vi "GenAppMainResize.vi"() -> ()   [LabVIEW 2018]
doc: "DESCRIPTION\nGeneral Application \n\nVERSION\nD1:00\nFirst Release To customer\nDD/MM/YYYY\n\nTemplate D2:01\nMade lighter and simpler\n14-04-2020"
uses:
  SubVIs/Controls/SetupModeState.ctl
  <vilib>/event_ctls.llb/eventsource.ctl
  SubVIs/Controls/DisplayQCommand.ctl
  SubVIs/Controls/QueueCommand.ctl
  SubVIs/Controls/DisplayMessage.ctl
  SubVIs/Controls/Transition.ctl
  SubVIs/utilities/Error/ErrorCommand.ctl
  SubVIs/Controls/Tab.ctl
  SubVIs/Controls/StateMessage.ctl
  SubVIs/Error/ErrorMessage.ctl
  SubVIs/utilities/Config/System Config Data Manager Parameter.ctl
  SubVIs/utilities/Config/ConfigCommand.ctl
panel:
  out "Time":string
  out "Version":string
  out "State":T1=enum."Initialising"
  out "Error":string
  out "ErrorIndicator":bool
  in  "ViewError":bool
  in  "Main Screen Tabs":enum32{"Main Screen"}(tab)
  out "Tab Control":T2(tab)
  out "ConfigdB path":path
  in  "ErrorLog":i32(listbox)
  in  "ButtonTabs":enum32{"Normal", "Error"}(tab)
  in  "Clear Alarm":bool
  in  "ErrorLog 2":bool
  in  "Home Button":bool
  in  "Error Loop":enum16{"Event Loop", "UI Q Loop", "State Loop"}(ring)
  in  "Generate Error":bool
  out "ErrorHandlingLoop":i32
  out "StateMachineLoop":i32
  out "UILoop":i32
  out "EventLoop":i32
  in  "Enter Password":string
  out "EngMode?":bool
  out "Status":string
  in  "Source":T3 items=["LabVIEW UI"=0, "ActiveX"=1, "User Event"=25]
  in  "exit":bool
  in  "Stop":bool
  in  "Start":bool
  # "GenAppMainResize"
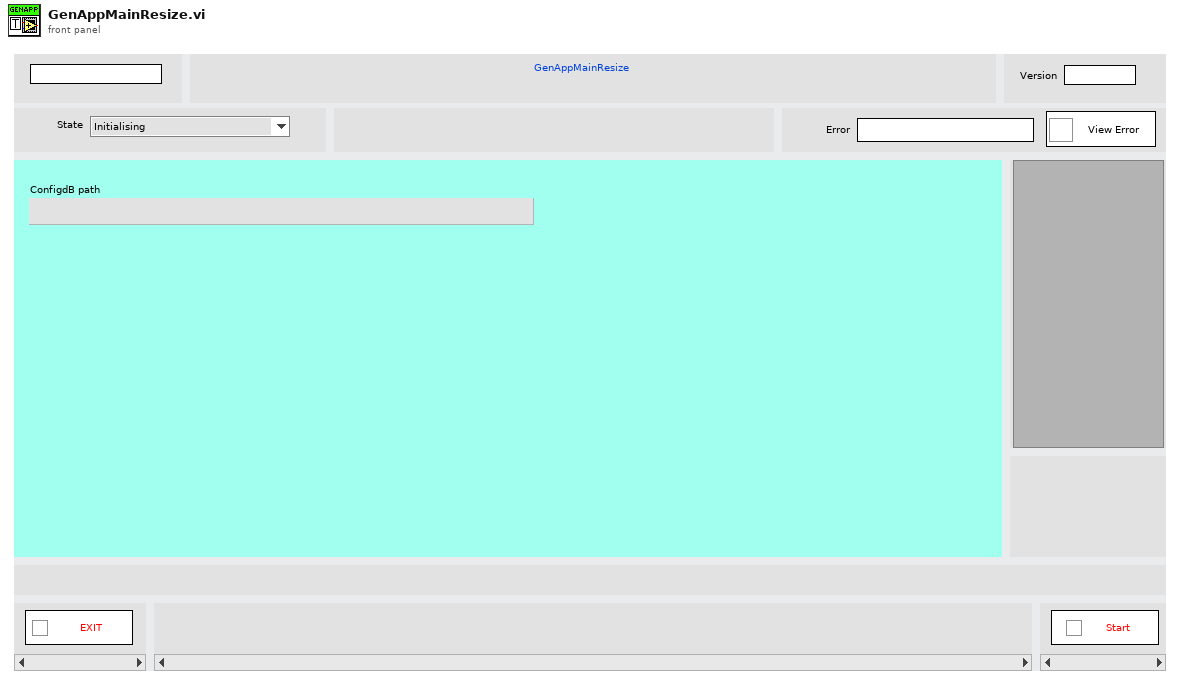
[diagram p1: front panel]
types:
  T1 = typedef "SetupModeState.ctl" = enum16{"No State - Error", "Initialising", "Idling", "Running", "Erroring", "Exiting"}
  T2 = enum32{"Welcome Screen", "Eng Set Up", "Oppo Run Screen", "Eng Run Screen", "Test Report Screen", "Error"}
  T3 = typedef "eventsource.ctl" = u32
  T4 = typedef "DisplayQCommand.ctl" = enum16{"No Command - Error", "Initialise", "Get Q Reference", "Add Item to Bottom", "Add Item to Top", "Flush Q", "Dequeue", "Peek Next Element", "Close"}
  T5 = typedef "QueueCommand.ctl" = enum16{"No Command - Error", "Initialise", "Add to Bottom", "Add To Top", "Get Ref", "Close"}
  T6 = typedef "ErrorCommand.ctl" = enum16{"No Command - Error", "Set to Dev Mode", "Set To Released Mode", "Set Error", "Log Error", "Throw Error", "Log & Throw Error", "Set Error Timed"}
  T7 = enum32{"invalid app kind", "Development System", "Run Time System", "Student Edition", "Embedded LabVIEW", "Evaluation", "Custom"}
  T8 = typedef "DisplayMessage.ctl" = enum16{"No Message - Ignore", "Display Message", "Set Tab", "Set Status", "Add Error Message", "Clear Error History", "Generate Error", "Set Idling Display", "Set Running Display", "Stop"}
  T9 = typedef "ErrorMessage.ctl" = enum16{"No Message - Ignore", "Display Message", "Stop"}
  T10 = typedef "StateMessage.ctl" = cluster{"Transition":T11, "variant":variant}
  T11 = typedef "Transition.ctl" = enum16{"No Transition - Error", "Initialise", "Login", "Authenticate", "Log on Fail", "Login Success", "Logout", "Generate Error", "Start", "Stop", "Exit"}
  T12 = typedef "ConfigCommand.ctl" = enum16{"No Command - Error", "Initialise Config SQLite", "Save Config", "Get Key", "Set Key", "Update Key", "Get Latest Config Data", "Get Config Data for Version", "Get Default Config Data"}
  T13 = typedef "System Config Data Manager Parameter.ctl" = enum16{"Eng Password", "DSN Connection", "User Password", "RunStatus", "InitialDataPath", "helpFilePath", "ErrorFilepath", "DatalogPath", "Hello"}
  T14 = typedef "Tab.ctl" = enum32{"Welcome Screen", "Eng Set Up", "Oppo Run Screen", "Eng Run Screen", "Test Report Screen", "Error"}
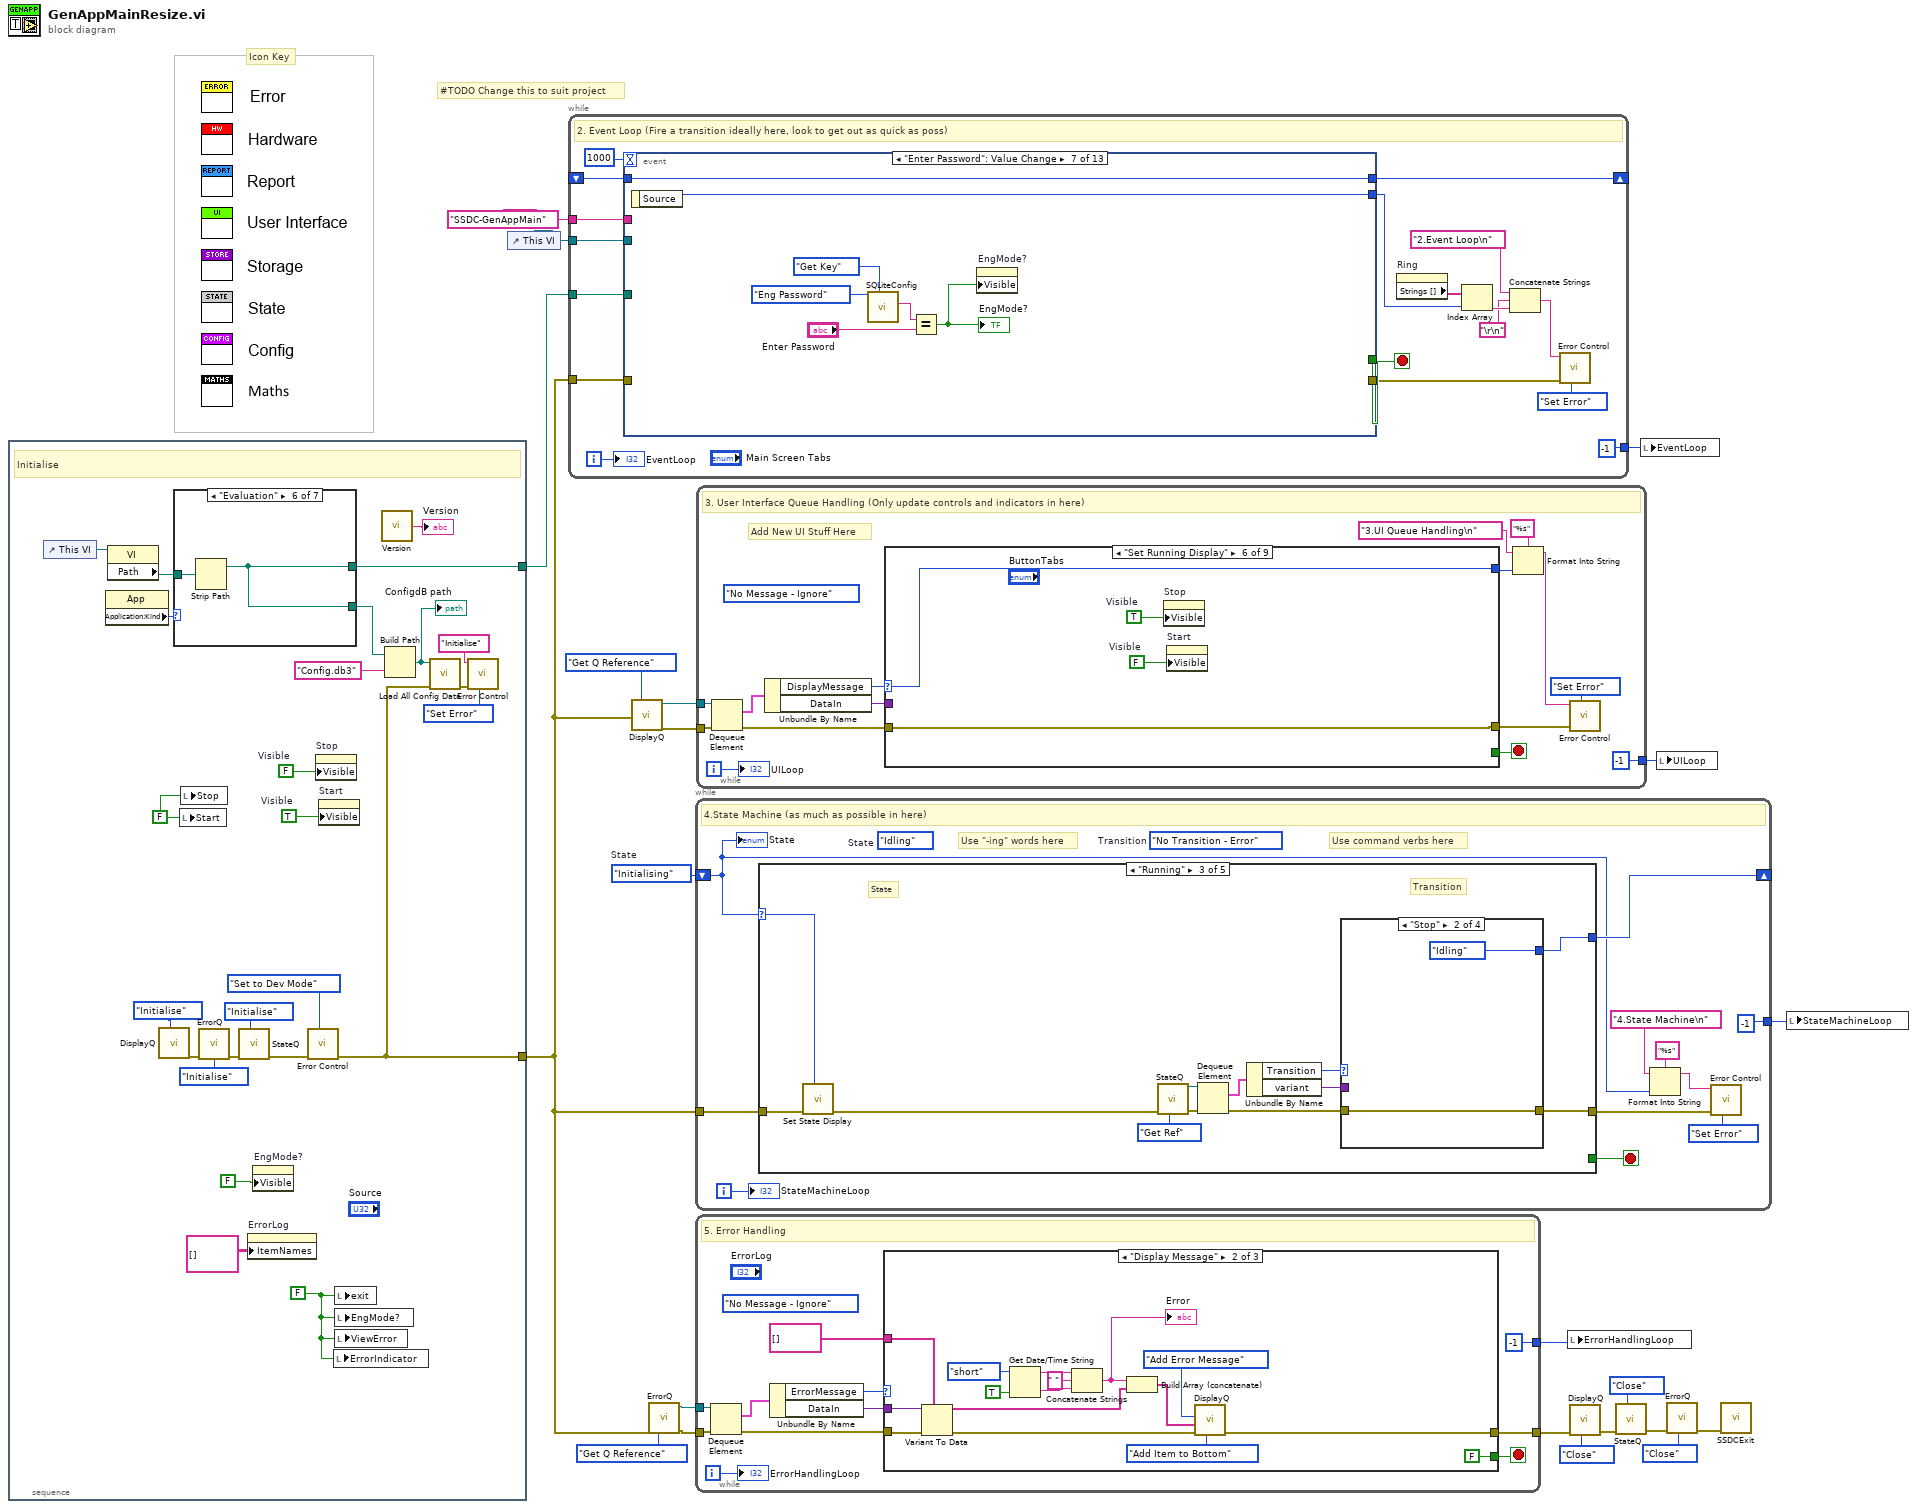
[diagram p0: block diagram]
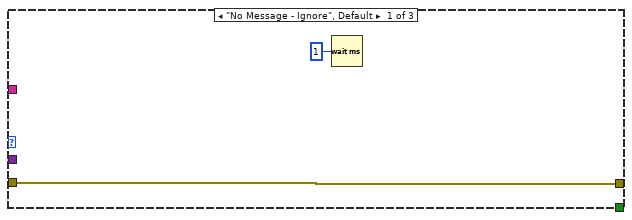
[diagram p2: hidden frame]
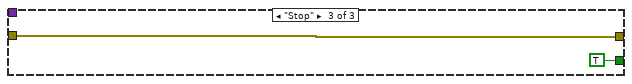
[diagram p3: hidden frame]
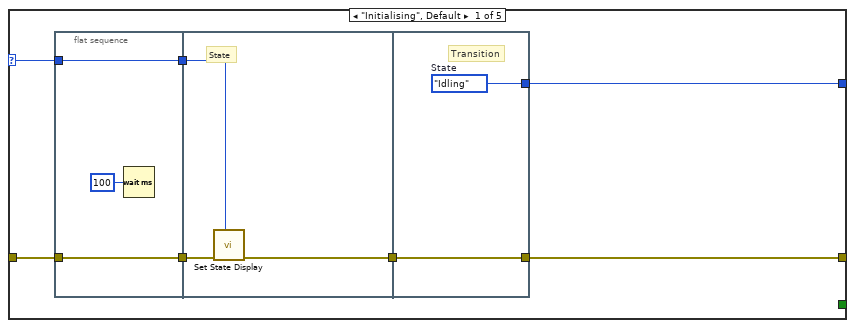
[diagram p4: hidden frame]
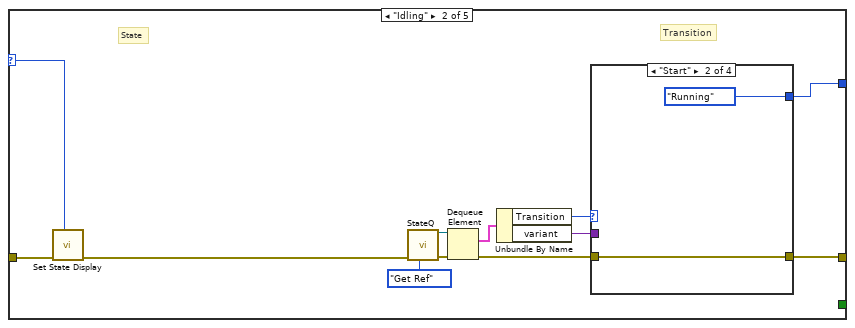
[diagram p5: hidden frame]
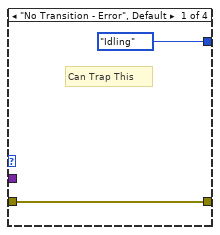
[diagram p6: hidden frame]
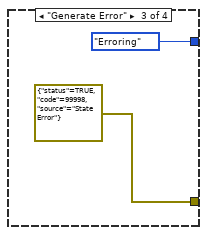
[diagram p7: hidden frame]
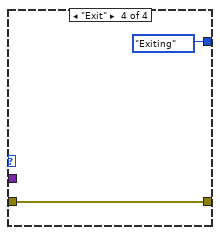
[diagram p8: hidden frame]
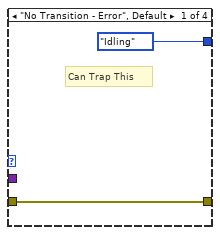
[diagram p9: hidden frame]
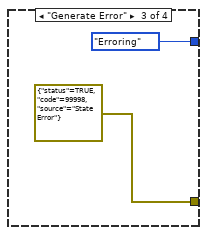
[diagram p10: hidden frame]
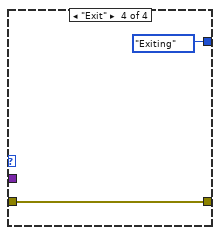
[diagram p11: hidden frame]
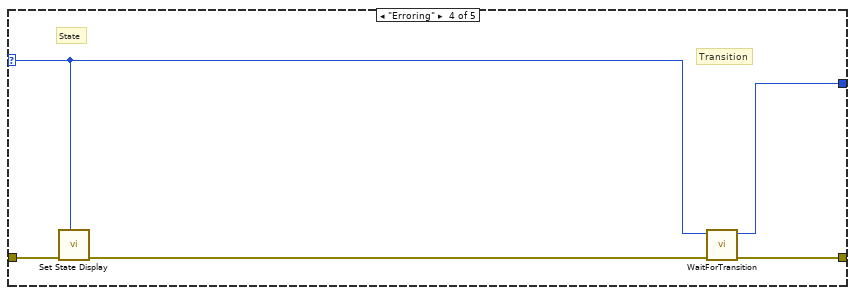
[diagram p12: hidden frame]
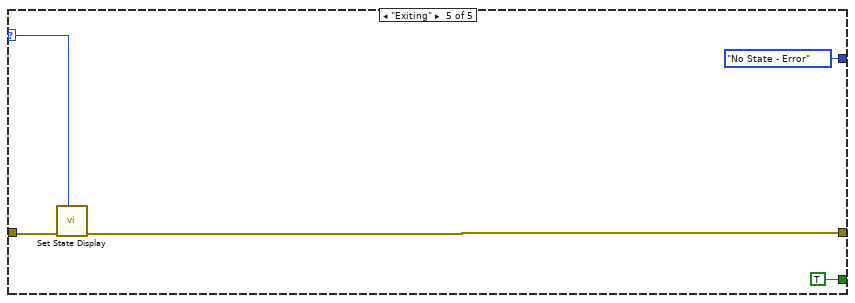
[diagram p13: hidden frame]
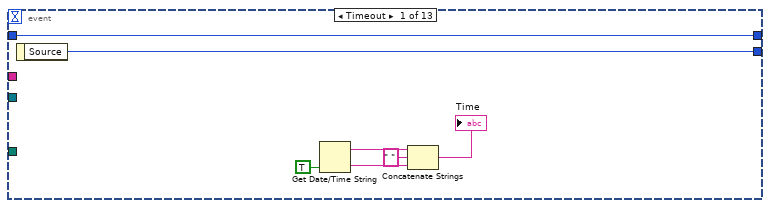
[diagram p14: hidden frame]
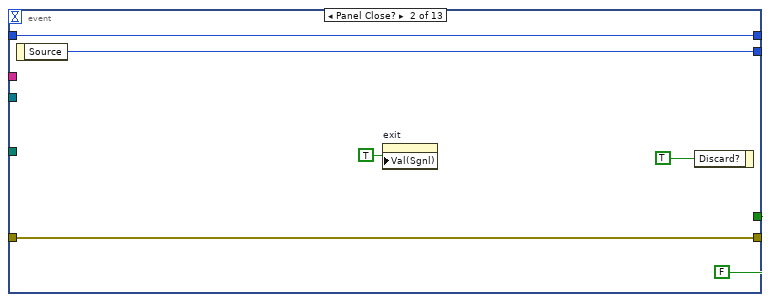
[diagram p15: hidden frame]
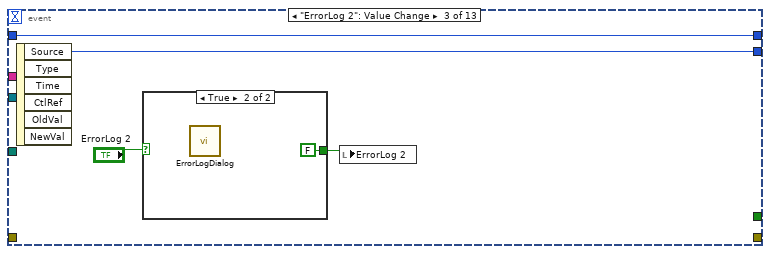
[diagram p16: hidden frame]
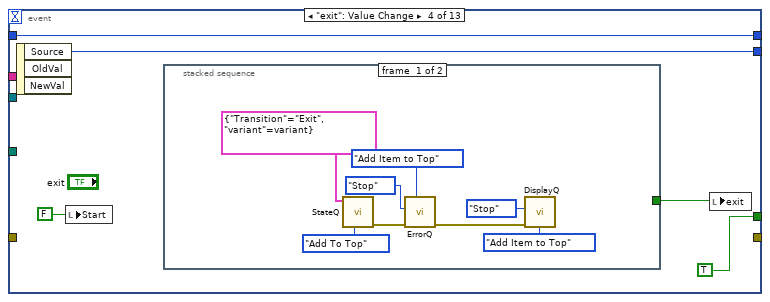
[diagram p18: hidden frame]
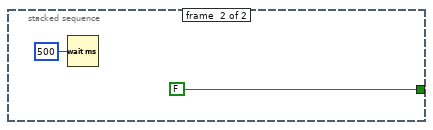
[diagram p19: hidden frame]
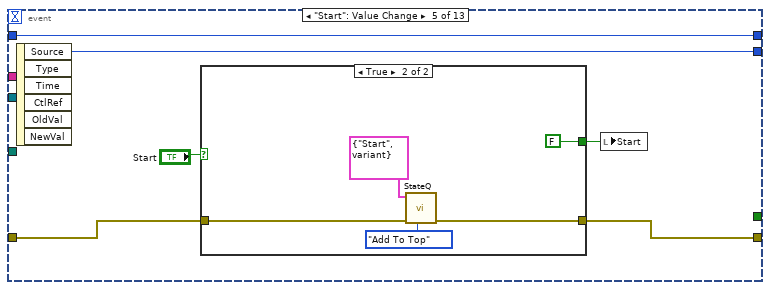
[diagram p20: hidden frame]
diagram:
  w22 = SetupModeState."Initialising"  # State
  # "#TODO Change this to suit project"
  # "Icon Key"
  n1 = stacked-sequence "1. Initialisation" {
    tunnel: [w26] -> w8
    tunnel: [w31] -> w16
    frame #0 {
      w24 = FALSE  # Visible
      w23 = TRUE  # Visible
      w29 = FALSE ("Stopped")
      w25 = FALSE ("Start")
      # "Initialise"
      n2 = control-ref of="This VI"() -> (w42:refnum<vi>)
      n3 = property class="App"() -> ("Application:Kind"=w41:T7)  [unwired: 2 in, 2 out]
      n4 = property class="VI"(reference=w42) -> ("Path"=w43:path)  [unwired: 1 in, 2 out]
      n5 = call "DisplayQ.vi"("command"=DisplayQCommand."Initialise") -> ("error out"=w36:errorcluster)  [unwired: 4 in, 3 out]
      n6 = case shown="\"Evaluation\"" w41 {
        tunnel: w43 -> [w48 w50 w54 w57 w59 w61 w63]
        tunnel: [w48 w49 w53 w56 w58 w60 w62] -> w32
        tunnel: [w48 w49 w51 w56 w58 w60 w62] -> w31
        frame "invalid app kind", Default {
        }
        frame "Development System" {
          n7 = Strip Path(path=w50) -> (stripped path=w49:path)  [unwired: 1 out]
        }
        frame "Run Time System" {
          n8 = Strip Path(path=w54) -> (stripped path=w55:path)  [unwired: 1 out]
          n9 = Strip Path(path=w55) -> (stripped path=w51:path)  [unwired: 1 out]
          n10 = Build Path(base path=w51, name or relative path="data") -> (appended path=w53:path)
        }
        frame "Student Edition" {
          n11 = Strip Path(path=w57) -> (stripped path=w56:path)  [unwired: 1 out]
        }
        frame "Embedded LabVIEW" {
          n12 = Strip Path(path=w59) -> (stripped path=w58:path)  [unwired: 1 out]
        }
        frame "Evaluation" {
          n13 = Strip Path(path=w61) -> (stripped path=w60:path)  [unwired: 1 out]
        }
        frame "Custom" {
          n14 = Strip Path(path=w63) -> (stripped path=w62:path)  [unwired: 1 out]
        }
      }
      n15 = local write "Start"(w25) -> ()
      n16 = local write "Stop"(w25) -> ()
      n17 = call "ErrorQ.vi"("command"=DisplayQCommand."Initialise", "error in (no error)"=w36) -> ("error out"=w37:errorcluster)  [unwired: 3 in, 3 out]
      n18 = call "StateQ.vi"("QueueCommand"=QueueCommand."Initialise", "error in (no error)"=w37) -> ("error out"=w27:errorcluster)  [unwired: 5 in, 1 out]
      n19 = property on="ErrorLog" class="MCListbox (strict)"("ItemNames"=string[][] [] ("Item Names")) -> ()  [unwired: 2 in, 2 out]
      n20 = property on="EngMode?" class="Bool (strict)"("Visible"=FALSE) -> ()  [unwired: 2 in, 2 out]
      n21 = call "Error Control.vi"("Command"=ErrorCommand."Set to Dev Mode", "error in (no error)"=w27) -> ("error out"=w26:errorcluster)  [unwired: 6 in]
      n22 = property on="Stop" class="Bool (strict)"("Visible"=w24) -> ()  [unwired: 2 in, 2 out]
      n23 = property on="Start" class="Bool (strict)"("Visible"=w23) -> ()  [unwired: 2 in, 2 out]
      n24 = local write "ErrorIndicator"(w29) -> ()
      n25 = local write "exit"(w29) -> ()
      n26 = local write "EngMode?"(w29) -> ()
      n27 = local write "ViewError"(w29) -> ()
      n28 = call "Version.vi"() -> ("Version"=→"Version":string)  [unwired: 5 in]
      n29 = Build Path(base path=w32, name or relative path="Config.db3") -> (appended path=w44:path)
      "ConfigdB path" <- w44
      n30 = call "Load All Config Data.vi"("error in (no error)"=w26, "path"=w44) -> ("error out"=w34:errorcluster)  [unwired: 5 in]
      n31 = call "Error Control.vi"("Command"=ErrorCommand."Set Error", "error in (no error)"=w34, "Source"="Initialise") -> ()  [unwired: 5 in, 1 out]
    }
  }
  n32 = control-ref of="This VI"() -> (w21:refnum<vi>)
  n33 = while "2. Event Loop" {
    tunnel: w8 -> [w78]
    shift-right: [w73] -> _
    shift-left: _ -> [w72]
    tunnel: w21 -> [w67]
    tunnel: [-1 ("ErrorHandlingLoop")] -> w17
    tunnel: w16 -> [w65]
    tunnel: "SSDC-GenAppMain" ("name or relative path") -> [w64]
    i -> [w81]
    stop <- w80 stop-if-true
    # "2. Event Loop (Fire a transition ideally here, look to get out as quick as poss)"
    n34 = event shown="[6] \"Enter Password\": Value Change" {
      selector: _ -> [_ _ _ _ _ _ _ _ _ _ _ _ _]
      dyn-events: _ -> [_ _ _ _ _ _ _ _ _ _ _ _ _]
      timeout: 1000 -> [_ _ _ _ _ _ _ _ _ _ _ _ _]
      tunnel: [_ FALSE ("STOP?") _ TRUE ("STOP?") _ _ _ w152 _ _ _ _ _] -> w80
      tunnel: w78 -> [_ w91 _ _ w116 w129 _ w148 w168 w184 w195 w216 _]
      tunnel: [_ w91 _ _ w115 w128 _ w147 w167 w183 w194 w215 _] -> w76
      tunnel: [w83 w90 w98 w101 w120 w132 w139 w150 w162 w182 w190 w211 w229] -> w74
      tunnel: [w82 w89 w97 w100 w119 w131 w140 w151 w163 w181 w191 w217 w230] -> w73
      tunnel: w72 -> [w82 w89 w97 w100 w119 w131 w140 w151 _ w181 w191 w217 w230]
      tunnel: w67 -> [_ _ _ _ _ _ _ w149 _ _ _ _ w228]
      tunnel: w65 -> [_ _ _ _ _ _ _ w146 _ _ _ _ _]
      tunnel: w64 -> [_ _ _ _ _ _ _ _ _ _ _ _ _]
      event Timeout {
        n35 = event-data() -> ("Source"=w83:T3)  [unwired: 1 in]
        n36 = Get Date/Time String(want seconds? (F)=TRUE) -> (date string=w87:string, time string=w86:string)  [unwired: 2 in]
        n37 = Concatenate Strings(w87, " " ("string"), w86) -> (→"Time":string)
      }
      event Panel Close? {
        n38 = event-data() -> ("Source"=w90:T3)  [unwired: 1 in]
        n39 = property on="exit" class="Bool (strict)"("Val(Sgnl)"=TRUE ("Value (Signaling)")) -> ()  [unwired: 2 in, 2 out]
        n40 = event-data("Discard?"=TRUE) -> ()  [unwired: 1 in, 1 out]
      }
      event "ErrorLog 2": Value Change {
        n41 = event-data() -> ("Source"=w98:T3)  [unwired: 1 in, 5 out]
        n42 = case shown="True" "ErrorLog 2" {
          tunnel: [_ FALSE] -> w95
          frame False {
          }
          frame True {
            n43 = call "ErrorLogDialog.vi"() -> ()  [unwired: 11 in, 1 out]
          }
        }
        n44 = local write "ErrorLog 2"(w95) -> ()
      }
      event "exit": Value Change {
        n45 = event-data() -> ("Source"=w101:T3)  [unwired: 1 in, 2 out]
        n46 = local write "Start"(FALSE ("Start")) -> ()
        n47 = stacked-sequence {
          tunnel: [_ FALSE] -> w102
          frame #0 {
            n48 = call "StateQ.vi"("QueueCommand"=QueueCommand."Add To Top", "output cluster"=T10 {"Transition"=enum."Exit", "variant"=variant}) -> ("error out"=w109:errorcluster)  [unwired: 5 in, 1 out]
            n49 = call "ErrorQ.vi"("command"=DisplayQCommand."Add Item to Top", "error in (no error)"=w109, "ErrorMessage"=ErrorMessage."Stop") -> ("error out"=w106:errorcluster)  [unwired: 2 in, 3 out]
            n50 = call "DisplayQ.vi"("command"=DisplayQCommand."Add Item to Top", "error in (no error)"=w106, "DisplayMessage"=DisplayMessage."Stop") -> ()  [unwired: 2 in, 4 out]
          }
          frame #1 {
            n51 = Wait (ms)(milliseconds to wait=u32 500) -> ()  [unwired: 1 out]
          }
        }
        n52 = local write "exit"(w102) -> ()
      }
      event "Start": Value Change {
        n53 = event-data() -> ("Source"=w120:T3)  [unwired: 1 in, 5 out]
        n54 = case shown="True" "Start" {
          tunnel: [_ FALSE ("Start")] -> w117
          tunnel: w116 -> [w121 w123]
          tunnel: [w121 w122] -> w115
          frame False {
          }
          frame True {
            n55 = call "StateQ.vi"("QueueCommand"=QueueCommand."Add To Top", "error in (no error)"=w123, "output cluster"=T10 {"Transition"=enum."Start", "variant"=variant}) -> ("error out"=w122:errorcluster)  [unwired: 4 in, 1 out]
          }
        }
        n56 = local write "Start"(w117) -> ()
      }
      event "Stop": Value Change {
        n57 = event-data() -> ("Source"=w132:T3)  [unwired: 1 in, 5 out]
        n58 = case shown="True" "Stop" {
          tunnel: [_ FALSE ("Start")] -> w130
          tunnel: w129 -> [w133 w135]
          tunnel: [w133 w134] -> w128
          frame False {
          }
          frame True {
            n59 = call "StateQ.vi"("QueueCommand"=QueueCommand."Add To Top", "error in (no error)"=w135, "output cluster"=T10 {"Transition"=enum."Stop", "variant"=variant}) -> ("error out"=w134:errorcluster)  [unwired: 4 in, 1 out]
          }
        }
        n60 = local write "Stop"(w130) -> ()
      }
      event "Enter Password": Value Change {
        n61 = event-data() -> ("Source"=w139:T3)  [unwired: 1 in]
        n62 = call "SQLiteConfig.vi"("ConfigCommand"=ConfigCommand."Get Key", "Parameter"=System_Config_Data_Manager_Parameter."Eng Password") -> ("KeyData"=w141:string)  [unwired: 3 in, 3 out]
        n63 = Equal?(x=w141, y="Enter Password") -> (x = y?=w145:bool)
        "EngMode?" <- w145
        n64 = property on="EngMode?" class="Bool (strict)"("Visible"=w145) -> ()  [unwired: 2 in, 2 out]
      }
      event Menu Selection (User) {
        n65 = event-data() -> ("Source"=w150:T3, "ItemTag"=w153:string)  [unwired: 1 in]
        n66 = case shown="\"About\"" w153 {
          tunnel: [_ FALSE _ _] -> w152
          tunnel: w149 -> [_ _ _ w161]
          tunnel: w148 -> [w154 w155 w158 w159]
          tunnel: [w154 w155 w158 w159] -> w147
          tunnel: w146 -> [_ _ _ _]
          frame "False", Default {
          }
          frame "Exit" {
            n67 = property on="exit" class="Bool (strict)"("Val(Sgnl)"=TRUE ("Value (Signaling)")) -> ()  [unwired: 2 in, 2 out]
          }
          frame "Configuration" {
            n68 = call "ConfigSQLiteSettingDialog.vi"() -> ()  [unwired: 1 in]
          }
          frame "About" {
            n69 = property class="VI"(reference=w161) -> ("Description"=w160:string)  [unwired: 1 in, 2 out]
            n70 = call "AboutScreen.vi"("Version Info. In"=w160) -> ()  [unwired: 11 in]
          }
        }
      }
      event "ViewError": Value Change {
        n71 = event-data() -> ("Source"=w162:T3)  [unwired: 1 in]
        n72 = local read "Tab Control"() -> (w164:T2)
        n73 = case shown="True" "ViewError" {
          tunnel: w168 -> [w171 w175]
          tunnel: [w171 w174] -> w167
          tunnel: [FALSE FALSE] -> w165
          tunnel: w164 -> [w169 w172]
          tunnel: [w169 w172] -> w163
          frame False {
          }
          frame True {
            n74 = call "DisplayQ.vi"("command"=DisplayQCommand."Add Item to Bottom", "error in (no error)"=w175, "DataIn"=Tab."Error" ("Tab Control"), "DisplayMessage"=DisplayMessage."Set Tab") -> ("error out"=w174:errorcluster)  [unwired: 1 in, 3 out]
          }
        }
        n75 = local write "ViewError"(w165) -> ()
      }
      event "Clear Alarm": Value Change {
        n76 = event-data() -> ("Source"=w182:T3)  [unwired: 1 in]
        n77 = case shown="True" "Clear Alarm" {
          tunnel: w184 -> [w186 w188]
          tunnel: [w186 w188] -> w183
          tunnel: [FALSE FALSE] -> w179
          frame False {
          }
          frame True {
            n78 = local write "ErrorIndicator"(FALSE ("ErrorIndicator")) -> ()
          }
        }
        n79 = local write "Clear Alarm"(w179) -> ()
      }
      event "Home Button": Value Change {
        n80 = event-data() -> ("Source"=w190:T3)  [unwired: 1 in]
        n81 = case shown="True" "Home Button" {
          tunnel: w195 -> [w197 w202]
          tunnel: [w197 w201] -> w194
          tunnel: [FALSE FALSE] -> w193
          tunnel: w191 -> [_ w199]
          frame False {
          }
          frame True {
            n82 = case shown="\"Error\"" w199 {
              tunnel: [Tab."Welcome Screen" ("Tab Control") Tab."Oppo Run Screen" ("Tab Control") Tab."Eng Run Screen" ("Tab Control") Tab."Test Report Screen" ("Tab Control") Tab."Error" ("Tab Control") Tab."Eng Run Screen" ("Tab Control")] -> w198
              frame "Welcome Screen" {
              }
              frame "Oppo Run Screen" {
              }
              frame "Eng Run Screen" {
              }
              frame "Test Report Screen" {
              }
              frame "Error" {
              }
              frame "Eng Set Up" {
              }
            }
            n83 = call "DisplayQ.vi"("command"=DisplayQCommand."Add Item to Bottom", "error in (no error)"=w202, "DataIn"=w198, "DisplayMessage"=DisplayMessage."Set Tab") -> ("error out"=w201:errorcluster)  [unwired: 1 in, 3 out]
          }
        }
        n84 = local write "Home Button"(w193) -> ()
      }
      event "Generate Error": Value Change {
        n85 = event-data() -> ("Source"=w211:T3)  [unwired: 1 in]
        n86 = case shown="\"UI Q Loop\"" "Error Loop" {
          tunnel: w216 -> [_ w220 w225]
          tunnel: [errorcluster {"status"=TRUE, "code"=99999, "source"="Random Event Error"} ("error out") w219 w226] -> w215
          tunnel: "Generate Error" -> [_ _ _]
          tunnel: [_ _ FALSE] -> w212
          frame "Event Loop", Default {
          }
          frame "UI Q Loop" {
            n87 = call "DisplayQ.vi"("command"=DisplayQCommand."Add Item to Bottom", "error in (no error)"=w220, "DisplayMessage"=DisplayMessage."Generate Error") -> ("error out"=w219:errorcluster)  [unwired: 2 in, 3 out]
          }
          frame "State Loop" {
            n88 = call "StateQ.vi"("QueueCommand"=QueueCommand."Add to Bottom", "error in (no error)"=w225, "output cluster"=T10 {"Transition"=enum."Generate Error", "variant"=variant}) -> ("error out"=w226:errorcluster)  [unwired: 4 in, 1 out]
          }
        }
        n89 = local write "Generate Error"(w212) -> ()
      }
      event "Version": Mouse Down {
        n90 = event-data() -> ("Source"=w229:T3)  [unwired: 1 in]
        n91 = property class="VI"(reference=w228) -> ("Description"=w231:string)  [unwired: 1 in, 2 out]
        n92 = call "VIDescription.vi"("VersionData In"=w231) -> ()  [unwired: 10 in, 1 out]
      }
    }
    n93 = property on="Ring" class="Ring (strict)"() -> ("Strings []"=w75:string[])  [unwired: 2 in, 2 out]
    n94 = Index Array(array=w75, index=w74) -> (element=w71:string)
    n95 = Concatenate Strings("2.Event Loop\n", "\r\n", w71) -> (w70:string)
    n96 = call "Error Control.vi"("Command"=ErrorCommand."Set Error", "error in (no error)"=w76, "Source"=w70) -> ()  [unwired: 5 in, 1 out]
    "EventLoop" <- w81
  }
  n97 = call "DisplayQ.vi"("command"=DisplayQCommand."Get Q Reference", "error in (no error)"=w8) -> ("error out"=w10:errorcluster, "queue out"=w11:refnum<queue>)  [unwired: 3 in, 2 out]
  n98 = call "ErrorQ.vi"("command"=DisplayQCommand."Get Q Reference", "error in (no error)"=w8) -> ("error out"=w13:errorcluster, "queue out"=w14:refnum<queue>)  [unwired: 3 in, 2 out]
  n99 = while {
    shift-right: [w240] -> _
    shift-left: w22 -> [w236]
    tunnel: w8 -> [w241]
    tunnel: [-1 ("ErrorHandlingLoop")] -> w19
    i -> [w239]
    stop <- w242 stop-if-true
    (unwired) SetupModeState."Idling"  # State
    (unwired) Transition."No Transition - Error"  # Transition
    # "Use command verbs here"
    # "Use \"-ing\" words here"
    # "4.State Machine (as much as possible in here)"
    n100 = case shown="\"Running\"" w236 {
      selector: w236 -> [w248 w268 w288 w298 w304]
      tunnel: [_ _ _ _ TRUE] -> w242
      tunnel: w241 -> [w249 w269 w289 w302 w305]
      tunnel: [w247 w259 w279 w301 SetupModeState."No State - Error" ("State 2")] -> w240
      tunnel: [w246 w260 w280 w300 w303] -> w237
      frame "Initialising", Default {
        n101 = flat-sequence {
          tunnel: w248 -> [w251]
          tunnel: w249 -> [w252]
          tunnel: [w252] -> w244
          tunnel: [w251] -> w243
          tunnel: [w253] -> w245
          tunnel: w244 -> [w255]
          tunnel: w243 -> [w254]
          tunnel: [w257] -> w247
          tunnel: [w256] -> w246
          tunnel: w245 -> [w256]
          frame #0 {
            n102 = Wait (ms)(milliseconds to wait=u32 100) -> ()  [unwired: 1 out]
          }
          frame #1 {
            # "State"
            n103 = call "Set State Display.vi"("State"=w254, "error in (no error)"=w255) -> ("error out"=w253:errorcluster)  [unwired: 6 in]
          }
          frame #2 {
            w257 = SetupModeState."Idling"  # State
            # "Transition"
          }
        }
      }
      frame "Idling" {
        # "Transition"
        # "State"
        n104 = call "Set State Display.vi"("State"=w268, "error in (no error)"=w269) -> ("error out"=w263:errorcluster)  [unwired: 6 in]
        n105 = call "StateQ.vi"("QueueCommand"=QueueCommand."Get Ref", "error in (no error)"=w263) -> ("error out"=w265:errorcluster, "queue out"=w264:refnum<queue>)  [unwired: 5 in]
        n106 = Dequeue Element(queue=w264, error in (no error)=w265) -> (element=w267:T10, error out=w262:errorcluster)  [unwired: 1 in, 2 out]
        n107 = Unbundle By Name(w267) -> ("Transition"=w261:T11, "variant"=w258:variant)
        n108 = case shown="\"Start\"" w261 {
          tunnel: [SetupModeState."Idling" ("State 2") SetupModeState."Running" ("State 2") SetupModeState."Erroring" ("State 2") SetupModeState."Exiting" ("State 2")] -> w259
          tunnel: w262 -> [w270 w272 _ w276]
          tunnel: [w270 w272 errorcluster {"status"=TRUE, "code"=99998, "source"="State Error"} ("error out") w276] -> w260
          tunnel: w258 -> [_ _ _ _]
          frame "No Transition - Error", Default {
            # "Can Trap This"
          }
          frame "Start" {
          }
          frame "Generate Error" {
          }
          frame "Exit" {
          }
        }
      }
      frame "Running" {
        # "Transition"
        # "State"
        n109 = call "Set State Display.vi"("State"=w288, "error in (no error)"=w289) -> ("error out"=w283:errorcluster)  [unwired: 6 in]
        n110 = call "StateQ.vi"("QueueCommand"=QueueCommand."Get Ref", "error in (no error)"=w283) -> ("error out"=w285:errorcluster, "queue out"=w284:refnum<queue>)  [unwired: 5 in]
        n111 = Dequeue Element(queue=w284, error in (no error)=w285) -> (element=w287:T10, error out=w282:errorcluster)  [unwired: 1 in, 2 out]
        n112 = Unbundle By Name(w287) -> ("Transition"=w281:T11, "variant"=w278:variant)
        n113 = case shown="\"Stop\"" w281 {
          tunnel: [SetupModeState."Idling" ("State 2") SetupModeState."Idling" ("State 2") SetupModeState."Erroring" ("State 2") SetupModeState."Exiting" ("State 2")] -> w279
          tunnel: w282 -> [w290 w292 _ w296]
          tunnel: [w290 w292 errorcluster {"status"=TRUE, "code"=99998, "source"="State Error"} ("error out") w296] -> w280
          tunnel: w278 -> [_ _ _ _]
          frame "No Transition - Error", Default {
            # "Can Trap This"
          }
          frame "Stop" {
          }
          frame "Generate Error" {
          }
          frame "Exit" {
          }
        }
      }
      frame "Erroring" {
        # "Transition"
        # "State"
        n114 = call "Set State Display.vi"("State"=w298, "error in (no error)"=w302) -> ("error out"=w299:errorcluster)  [unwired: 6 in]
        n115 = call "WaitForTransition.vi"("error in (no error)"=w299, "State"=w298) -> ("error out"=w300:errorcluster, "StateOut"=w301:T1)  [unwired: 4 in]
      }
      frame "Exiting" {
        n116 = call "Set State Display.vi"("State"=w304, "error in (no error)"=w305) -> ("error out"=w303:errorcluster)  [unwired: 6 in]
      }
    }
    n117 = Format Into String(format string="%s", initial string="4.State Machine\n", w236) -> (resulting string=w235:string)  [unwired: 1 in, 1 out]
    n118 = call "Error Control.vi"("Command"=ErrorCommand."Set Error", "error in (no error)"=w237, "Source"=w235) -> ()  [unwired: 5 in, 1 out]
    "StateMachineLoop" <- w239
    "State" <- w236
  }
  n119 = while {
    tunnel: w13 -> [w318]
    tunnel: w14 -> [w317]
    tunnel: [w309] -> w1
    tunnel: [-1 ("ErrorHandlingLoop")] -> w20
    i -> [w311]
    stop <- w312 stop-if-true
    (unwired) DisplayMessage."No Message - Ignore" ("DisplayMessage")
    # "5. Error Handling"
    n120 = Dequeue Element(queue=w317, error in (no error)=w318) -> (element=w316:cluster{"ErrorMessage":T9, "DataIn":variant}, error out=w313:errorcluster)  [unwired: 1 in, 2 out]
    n121 = Unbundle By Name(w316) -> ("ErrorMessage"=w314:T9, "DataIn"=w315:variant)
    n122 = case shown="\"Display Message\"" w314 {
      tunnel: w315 -> [_ w335 _]
      tunnel: w313 -> [w319 w334 w338]
      tunnel: [w319 w325 w338] -> w309
      tunnel: [_ FALSE ("STOP?") TRUE ("STOP?")] -> w312
      tunnel: string[] [] -> [_ w333 _]
      frame "No Message - Ignore", Default {
        n123 = Wait (ms)(milliseconds to wait=u32 1) -> ()  [unwired: 1 out]
      }
      frame "Display Message" {
        n124 = Variant To Data(error in=w334, type=w333, Variant=w335) -> (data=w327:string[], error out=w326:errorcluster)
        n125 = Get Date/Time String(date format (0)=enum16{"short", "long", "abbreviated"}."short", want seconds? (F)=TRUE) -> (date string=w330:string, time string=w329:string)  [unwired: 1 in]
        n126 = Concatenate Strings(w330, " " ("string"), w329) -> (w321:string)
        "Error" <- w321
        n127 = Build Array (concatenate)(w321, w327) -> (w322:string[])
        n128 = call "DisplayQ.vi"("command"=DisplayQCommand."Add Item to Bottom", "error in (no error)"=w326, "DataIn"=w322, "DisplayMessage"=DisplayMessage."Add Error Message") -> ("error out"=w325:errorcluster)  [unwired: 1 in, 3 out]
      }
      frame "Stop" {
      }
    }
    "ErrorHandlingLoop" <- w311
  }
  n129 = while "3. User Interface Queue Handling" {
    tunnel: w10 -> [w353]
    tunnel: w11 -> [w352]
    tunnel: [-1 ("ErrorHandlingLoop")] -> w18
    i -> [w344]
    stop <- w345 stop-if-true
    (unwired) DisplayMessage."No Message - Ignore" ("DisplayMessage")
    # "Add New UI Stuff Here"
    # "3. User Interface Queue Handling (Only update controls and indicators in here)"
    n130 = Dequeue Element(queue=w352, error in (no error)=w353) -> (element=w351:cluster{"DisplayMessage":T8, "DataIn":variant}, error out=w348:errorcluster)  [unwired: 1 in, 2 out]
    n131 = Unbundle By Name(w351) -> ("DisplayMessage"=w349:T8, "DataIn"=w350:variant)
    n132 = case shown="\"Set Running Display\"" w349 {
      selector: w349 -> [w354 w357 w360 w375 w382 w386 w390 w392 w394]
      tunnel: w350 -> [_ _ w369 w378 _ _ _ _ w398]
      tunnel: w348 -> [w355 w359 w362 w377 w381 w385 w389 _ w396]
      tunnel: [w355 w359 w361 w376 w381 w385 w389 errorcluster {"status"=TRUE, "code"=99997, "source"="UI Error"} ("error out") w395] -> w347
      tunnel: [_ TRUE ("STOP?") _ _ _ _ _ _ _] -> w345
      tunnel: [w354 w357 w360 w375 w382 w386 w390 w392 w394] -> w343
      frame "No Message - Ignore", Default {
        n133 = Wait (ms)(milliseconds to wait=u32 1) -> ()  [unwired: 1 out]
      }
      frame "Stop" {
      }
      frame "Display Message" {
        n134 = Variant To Data(error in=w362, type="" ("data"), Variant=w369) -> (data=w365:string, error out=w361:errorcluster)
        n135 = local read "State"() -> (w367:T1)
        n136 = Format Into String(w367) -> (resulting string=w366:string)  [unwired: 3 in, 1 out]
        n137 = Concatenate Strings(w366, " - " ("string"), w365) -> (→"Status":string)
      }
      frame "Add Error Message" {
        n138 = property on="ErrorLog" class="MCListbox (strict)"() -> ("ItemNames"=w373:string[][])  [unwired: 2 in, 2 out]
        n139 = Variant To Data(error in=w377, type=string[] [], Variant=w378) -> (data=w372:string[], error out=w376:errorcluster)
        n140 = Build Array (concatenate)(w373, w372) -> (w370:string[][])
        n141 = property on="ErrorLog" class="MCListbox (strict)"("ItemNames"=w370) -> ()  [unwired: 2 in, 2 out]
        "ErrorIndicator" <- TRUE ("ErrorIndicator")
      }
      frame "Set Idling Display" {
        w379 = FALSE  # Visible
        w380 = TRUE  # Visible
        n142 = property on="Stop" class="Bool (strict)"("Visible"=w379) -> ()  [unwired: 2 in, 2 out]
        n143 = property on="Start" class="Bool (strict)"("Visible"=w380) -> ()  [unwired: 2 in, 2 out]
      }
      frame "Set Running Display" {
        w383 = TRUE  # Visible
        w384 = FALSE  # Visible
        n144 = property on="Stop" class="Bool (strict)"("Visible"=w383) -> ()  [unwired: 2 in, 2 out]
        n145 = property on="Start" class="Bool (strict)"("Visible"=w384) -> ()  [unwired: 2 in, 2 out]
      }
      frame "Clear Error History" {
        n146 = property on="ErrorLog" class="MCListbox (strict)"("ItemNames"=string[][] []) -> ()  [unwired: 2 in, 2 out]
        n147 = local write "ErrorIndicator"(FALSE ("ErrorIndicator")) -> ()
      }
      frame "Generate Error" {
      }
      frame "Set Tab" {
        n148 = Variant To Data(error in=w396, type=Tab."Eng Run Screen" ("Tab Control"), Variant=w398) -> (data=→"Tab Control":T14, error out=w395:errorcluster)
      }
    }
    n149 = Format Into String(format string="%s", initial string="3.UI Queue Handling\n", w343) -> (resulting string=w342:string)  [unwired: 1 in, 1 out]
    n150 = call "Error Control.vi"("Command"=ErrorCommand."Set Error", "error in (no error)"=w347, "Source"=w342) -> ()  [unwired: 5 in, 1 out]
    "UILoop" <- w344
  }
  n151 = local write "ErrorHandlingLoop"(w20) -> ()
  n152 = call "DisplayQ.vi"("command"=DisplayQCommand."Close", "error in (no error)"=w1) -> ("error out"=w3:errorcluster)  [unwired: 3 in, 3 out]
  n153 = call "StateQ.vi"("QueueCommand"=QueueCommand."Close", "error in (no error)"=w3) -> ("error out"=w5:errorcluster)  [unwired: 5 in, 1 out]
  n154 = local write "EventLoop"(w17) -> ()
  n155 = local write "UILoop"(w18) -> ()
  n156 = call "ErrorQ.vi"("command"=DisplayQCommand."Close", "error in (no error)"=w5) -> ("error out"=w6:errorcluster)  [unwired: 3 in, 3 out]
  n157 = call "SSDCExit.vi"("error in (no error)"=w6) -> ()  [unwired: 6 in, 1 out]
  n158 = local write "StateMachineLoop"(w19) -> ()
